vi "IKsolver.vi"(9 "y":dbl, 10 "Arm Lengths":cluster{"L 1":dbl, "L 2":dbl, "L 4":dbl}, 11 "x":dbl) -> (3 "Angles(q)":dbl[](array[numeric]))   [LabVIEW 2024]
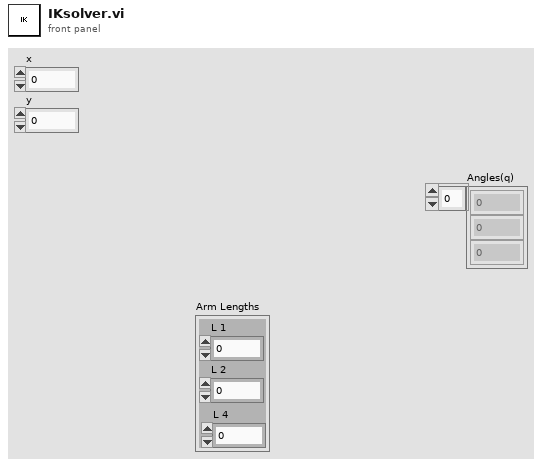
[diagram p1: front panel]
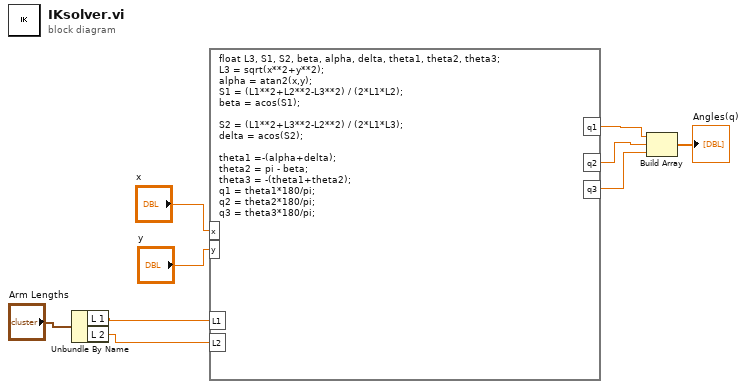
[diagram p0: block diagram]
diagram:
  n1 = Unbundle By Name("Arm Lengths") -> ("L 1"=w8:dbl, "L 2"=w7:dbl)
  n2 = formula code="float L3, S1, S2, beta, alpha, delta, theta1, theta2, theta3;\nL3 = sqrt(x**2+y**2);\nalpha = atan2(x,y);\nS1 = (L1**2+L2**2-L3**2) / (2*L1*L2);\nbeta = acos(S1);\n\nS2 = (L1**2+L3**2-L2**2) / (2*L1*L3);\ndelta = acos(S2);\n\ntheta1 =-(alpha+delta);\ntheta2 = pi - beta;\ntheta3 = -(theta1+theta2);\nq1 = theta1*180/pi;\nq2 = theta2*180/pi;\nq3 = theta3*180/pi;"("L1"=w8, "L2"=w7, "x"="x", "y"="y") -> ("q1"=w6:dbl, "q2"=w5:dbl, "q3"=w4:dbl)
  n3 = Build Array(w6, w5, w4) -> (→"Angles(q)":dbl[])
